vi "Validate Experiment Name.vi"(11 "Experiment Name":string) -> (2 "Error (if invalid)":string, 3 "Valid Experiment Name?":bool)   [LabVIEW 2020, in "RxnRover.lvlib" / "Experiment Manager.lvlib"]
uses:
  Experiment Manager.lvlib
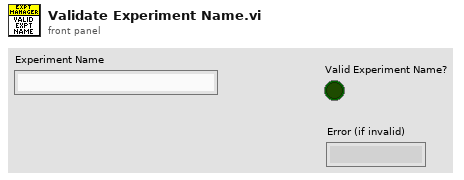
[diagram p1: front panel]
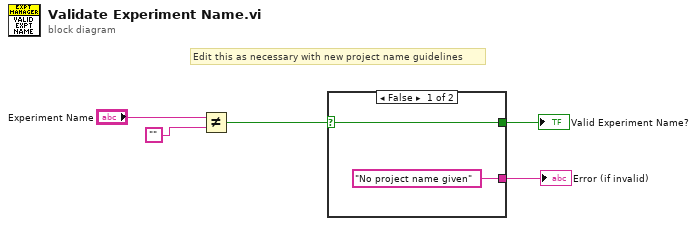
[diagram p0: block diagram]
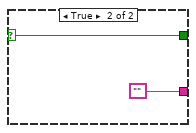
[diagram p2: hidden frame]
diagram:
  # "Edit this as necessary with new project name guidelines"
  n1 = Not Equal?(x="Experiment Name", y="") -> (x != y?=w3:bool)
  n2 = case shown="False" w3 {
    selector: w3 -> [w7 w9]
    tunnel: [w7 w9] -> w2
    tunnel: ["No project name given" ""] -> w1
    frame False {
    }
    frame True {
    }
  }
  "Valid Experiment Name?" <- w2
  "Error (if invalid)" <- w1
